vi "sanitize sql input.vi"(8 "error in":errorcluster, 10 "Sting in":string) -> (0 "error out":errorcluster, 1 "Ok?":bool=TRUE, 2 "String out":string)   [LabVIEW 2020, in "IDatabase.lvlib"]
uses:
  IDatabase/IDatabase.lvlib
  <vilib>/Utility/error.llb/Error Cluster From Error Code.vi
  <vilib>/regexp/Match Regular Expression.xnode
  <vilib>/ErrorRing/Error Ring.xnode
panel:
  # "Adapted from https://www.hiawatha-webserver.org/preventsqli\nthis vi uses match regex to filter out lazy and naive sql injection attacks"
  # "THIS WILL NOT PREVENT ALL SQL INJECTION.  YOU HAVE BEEN WARNED!"
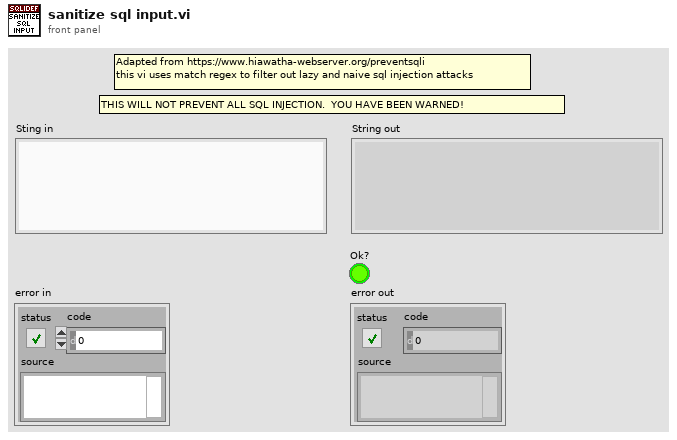
[diagram p1: front panel]
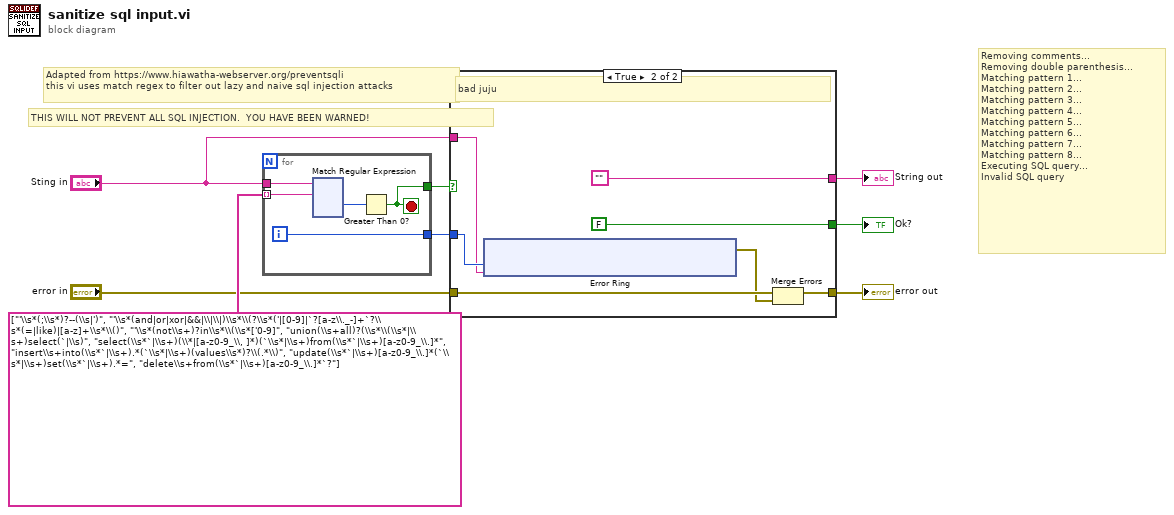
[diagram p0: block diagram]
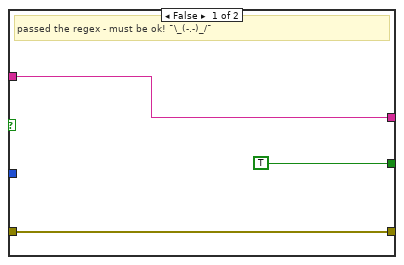
[diagram p2: hidden frame]
diagram:
  # "THIS WILL NOT PREVENT ALL SQL INJECTION.  YOU HAVE BEEN WARNED!"
  # "Removing comments...\nRemoving double parenthesis...\nMatching pattern 1...\nMatching pattern 2...\nMatching pattern 3...\nMatching pattern 4...\nMatching pattern 5...\nMatching pattern 6...\nMatching pattern 7...\nMatching pattern 8...\nExecuting SQL query...\nInvalid SQL query"
  # "Adapted from https://www.hiawatha-webserver.org/preventsqli\nthis vi uses match regex to filter out lazy and naive sql injection attacks"
  n1 = for {
    tunnel: "Sting in" -> [w13]
    tunnel: [w11] -> w6
    tunnel: string[] ["'\\s*(;\\s*)?--(\\s|')", "'\\s*(and|or|xor|&&|\\|\\|)\\s*\\(?\\s*('|[0-9]|`?[a-z\\._-]+`?\\s*(=|like)|[a-z]+\\s*\\()", "'\\s*(not\\s+)?in\\s*\\(\\s*['0-9]", "union(\\s+all)?(\\s*\\(\\s*|\\s+)select(`|\\s)", "select(\\s*`|\\s+)(\\*|[a-z0-9_\\, ]*)(`\\s*|\\s+)from(\\s*`|\\s+)[a-z0-9_\\.]*", "insert\\s+into(\\s*`|\\s+).*(`\\s*|\\s+)(values\\s*)?\\(.*\\)", "update(\\s*`|\\s+)[a-z0-9_\\.]*(`\\s*|\\s+)set(\\s*`|\\s+).*=", "delete\\s+from(\\s*`|\\s+)[a-z0-9_\\.]*`?"] -> [w10] mode=indexing
    tunnel: [w9] -> w7
    i -> [w11]
    stop <- w9 stop-if-true
    n2 = xnode "Match Regular Expression"("input string"=w13, "regular expression"=w10) -> ("offset past match"=w12:i32)  [unwired: 4 in, 4 out]
    n3 = Greater Than 0?(x=w12) -> (x > 0?=w9:bool)
  }
  n4 = case shown="True" w7 {
    tunnel: w6 -> [_ w135]
    tunnel: "Sting in" -> [w130 w134]
    tunnel: "error in" -> [w128 w133]
    tunnel: [w130 ""] -> w3
    tunnel: [TRUE FALSE] -> w2
    tunnel: [w128 w131] -> w1
    frame False {
      # "passed the regex - must be ok! ¯\\_(-.-)_/¯"
    }
    frame True {
      # "bad juju"
      n5 = xnode "Error Ring"("parameter 0"=w135, "parameter 1"=w134) -> ("error out"=w132:errorcluster)
      n6 = Merge Errors(w133, w132) -> (w131:errorcluster)
    }
  }
  "String out" <- w3
  "error out" <- w1
  "Ok?" <- w2
